vi "Set Magnet Field.vi"(4 "Mode":T2, 6 "Axis":T1, 8 "error in (no error)":errorcluster, 9 "Target Rate (T/min)":dbl, 10 "Target Field (T)":dbl, 11 "Instrument.Oxford1820 in":refnum<class "Instrument.OxfordVRM.lvclass">) -> (0 "error out":errorcluster, 3 "Instrument.Oxford1820 out":refnum<class "Instrument.OxfordVRM.lvclass">)   [LabVIEW 2016, in "Instrument.OxfordVRM.lvclass"]
uses:
  Instrument.OxfordVRM.lvclass
  <userlib>/LevyLab/Levylab Instruments/Instrument Types/Cryostat/Typedefs/Magnet Mode--Enum.ctl
  <userlib>/LevyLab/Levylab Instruments/Instrument Types/Cryostat/Typedefs/Magnet Axis--Enum.ctl
  Typedefs/Instrument.Oxford1820.Commands-enum.ctl
  Typedefs/Instrument.Oxford1820.setMagnet-cluster.ctl
  Typedefs/Targets.ctl
  <userlib>/LevyLab/Levylab Instruments/Instrument Types/Cryostat/Instrument.Cryostat.lvclass
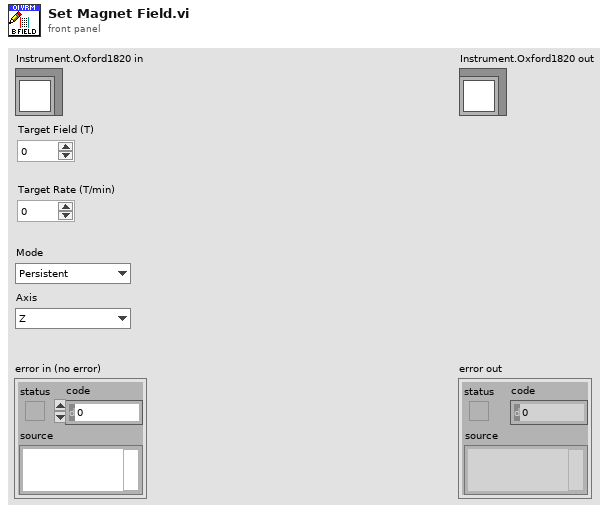
[diagram p1: front panel]
types:
  T1 = typedef "Instrument.Cryostat.lvclass/Magnet Axis--Enum.ctl" = enum16{"Z", "X", "Y"}
  T2 = typedef "Instrument.Cryostat.lvclass/Magnet Mode--Enum.ctl" = enum16{"Persistent", "Driven"}
  T3 = typedef "Instrument.OxfordVRM.lvclass/Instrument.Oxford1820.setMagnet-cluster.ctl" = cluster{"Target":T4, "persistent mode":bool}
  T4 = typedef "Instrument.OxfordVRM.lvclass/Targets.ctl" = cluster{"Field (T)":dbl, "Field Rate (T/min)":dbl}
  T5 = typedef "Instrument.OxfordVRM.lvclass/Instrument.Oxford1820.Commands-enum.ctl" = enum16{"setAction", "setTarget", "setSwitchHeat", "setLambda", "setFillMode", "setNeedleValve", "setMagnetField", "getStatus", "getTarget", "getSwitchHeat", "getPSUField", "newcommand", "getMagnetField"}
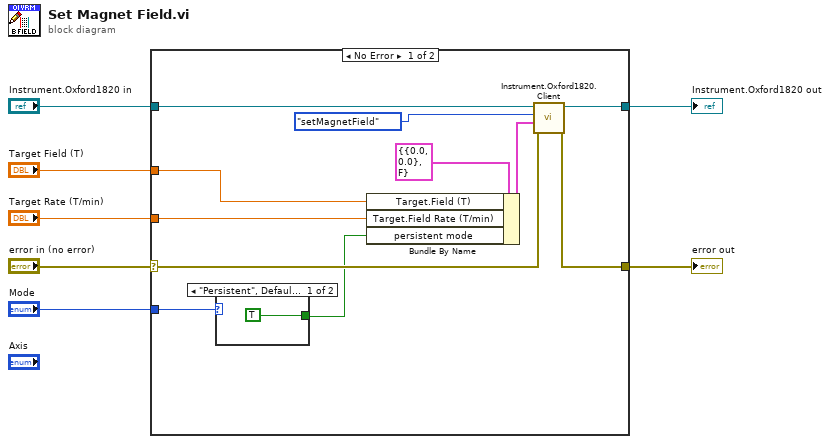
[diagram p0: block diagram]
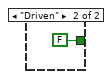
[diagram p2: hidden frame]
diagram:
  n1 = case shown="No Error" "error in (no error)" {
    selector: "error in (no error)" -> [w13 w22]
    tunnel: "Mode" -> [w18 _]
    tunnel: "Target Rate (T/min)" -> [w17 _]
    tunnel: [w12 w22] -> w5
    tunnel: "Target Field (T)" -> [w16 _]
    tunnel: "Instrument.Oxford1820 in" -> [w15 w21]
    tunnel: [w14 w21] -> w1
    frame No Error {
      n2 = case shown="\"Persistent\", Default" w18 {
        tunnel: [TRUE ("persistent mode") FALSE ("persistent mode")] -> w9
        frame "Persistent", Default {
        }
        frame "Driven" {
        }
      }
      n3 = Bundle By Name(cluster=T3 {"Target"={"Field (T)"=0.0, "Field Rate (T/min)"=0.0}, "persistent mode"=FALSE} ("output cluster"), "Target.Field (T)"=w16, "Target.Field Rate (T/min)"=w17, "persistent mode"=w9) -> (w10:T3)
      n4 = call "Instrument.Oxford1820.Client.vi"("error in (no error)"=w13, "Data"=w10, "Commands"=Instrument.Oxford1820.Commands-enum."setMagnetField", "Instrument.1820 in"=w15) -> ("error out"=w12:errorcluster, "Instrument.1820 out"=w14:refnum<class "Instrument.OxfordVRM.lvclass">)  [unwired: 5 in, 1 out]
    }
    frame Error {
    }
  }
  "Instrument.Oxford1820 out" <- w1
  "error out" <- w5
